vi "5-3Array_arrayoglu.vi"() -> ()   [LabVIEW 2024]
panel:
  out "max index(es)":i32[](array[numeric])
  out "max value 2":dbl
  out "transposed array":dbl[][](array[numeric])
  out "element 2":dbl
  in  "disabled index (col)":i32
  in  "index (row)":i32
  out "output array":dbl[](array[numeric])
  out "subarray":dbl[][](array[numeric])
  out "size(s) 2":i32[](array[numeric])
  in  "Array 8":dbl[][](array[numeric])
  out "Array 7":dbl[][](array[numeric])
  out "Array 6":dbl[](array[numeric])
  in  "length":i32
  in  "index 4":i32
  out "min value":i32
  out "max value":i32
  out "Array 5":dbl[](array[numeric])
  in  "new element/subarray 2":dbl
  in  "index 3":i32
  out "Array 4":dbl[](array[numeric])
  in  "new element/subarray":i32
  in  "index 2":i32
  in  "index":i32
  out "element":dbl
  out "size(s)":i32
  out "Array 3":dbl[](array[numeric])
  out "Array 2":dbl[](array[numeric])
  in  "dimension size":i32
  out "Array":dbl[](array[numeric])
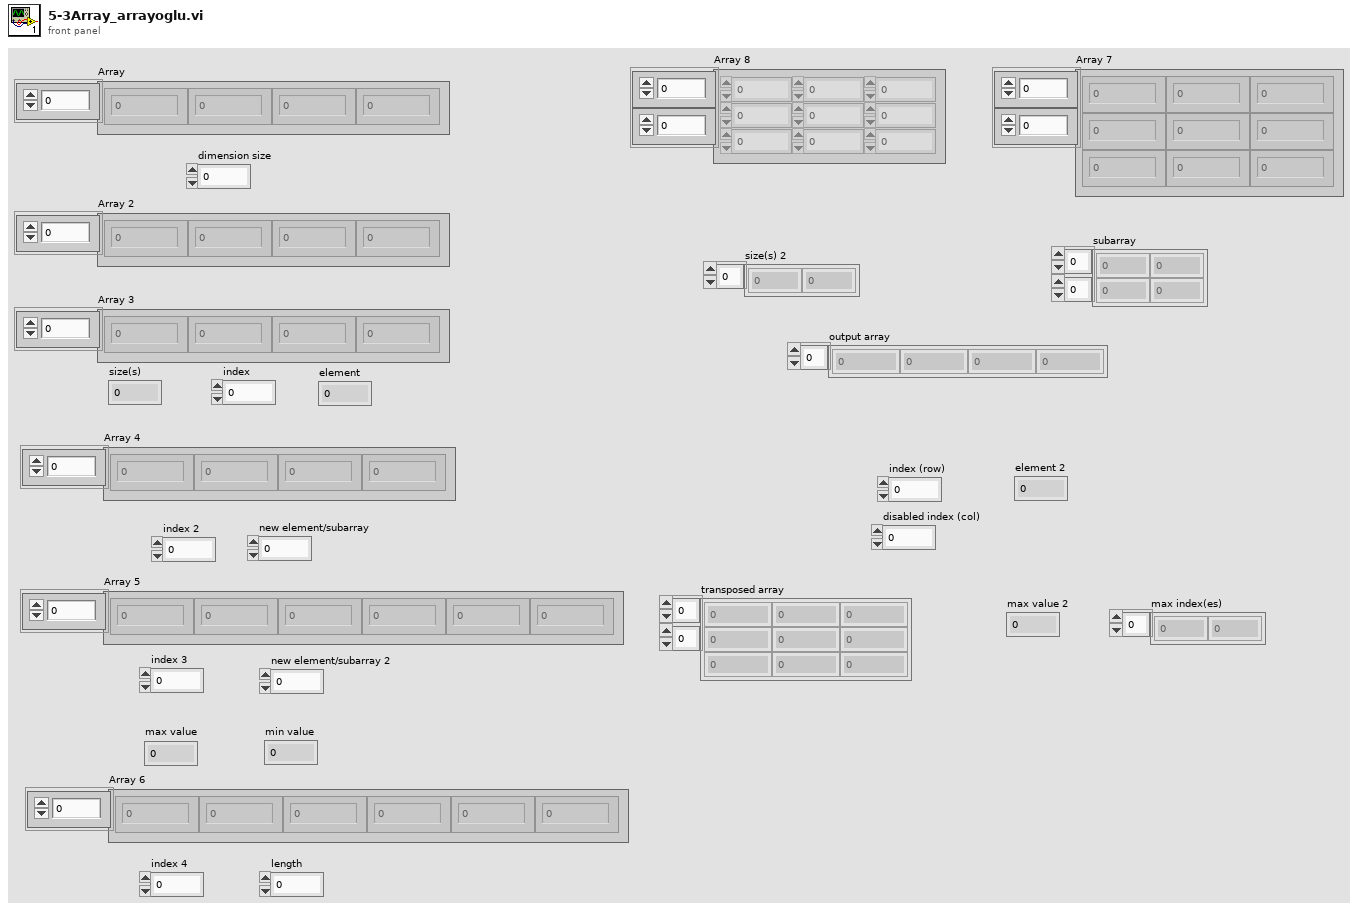
[diagram p1: front panel]
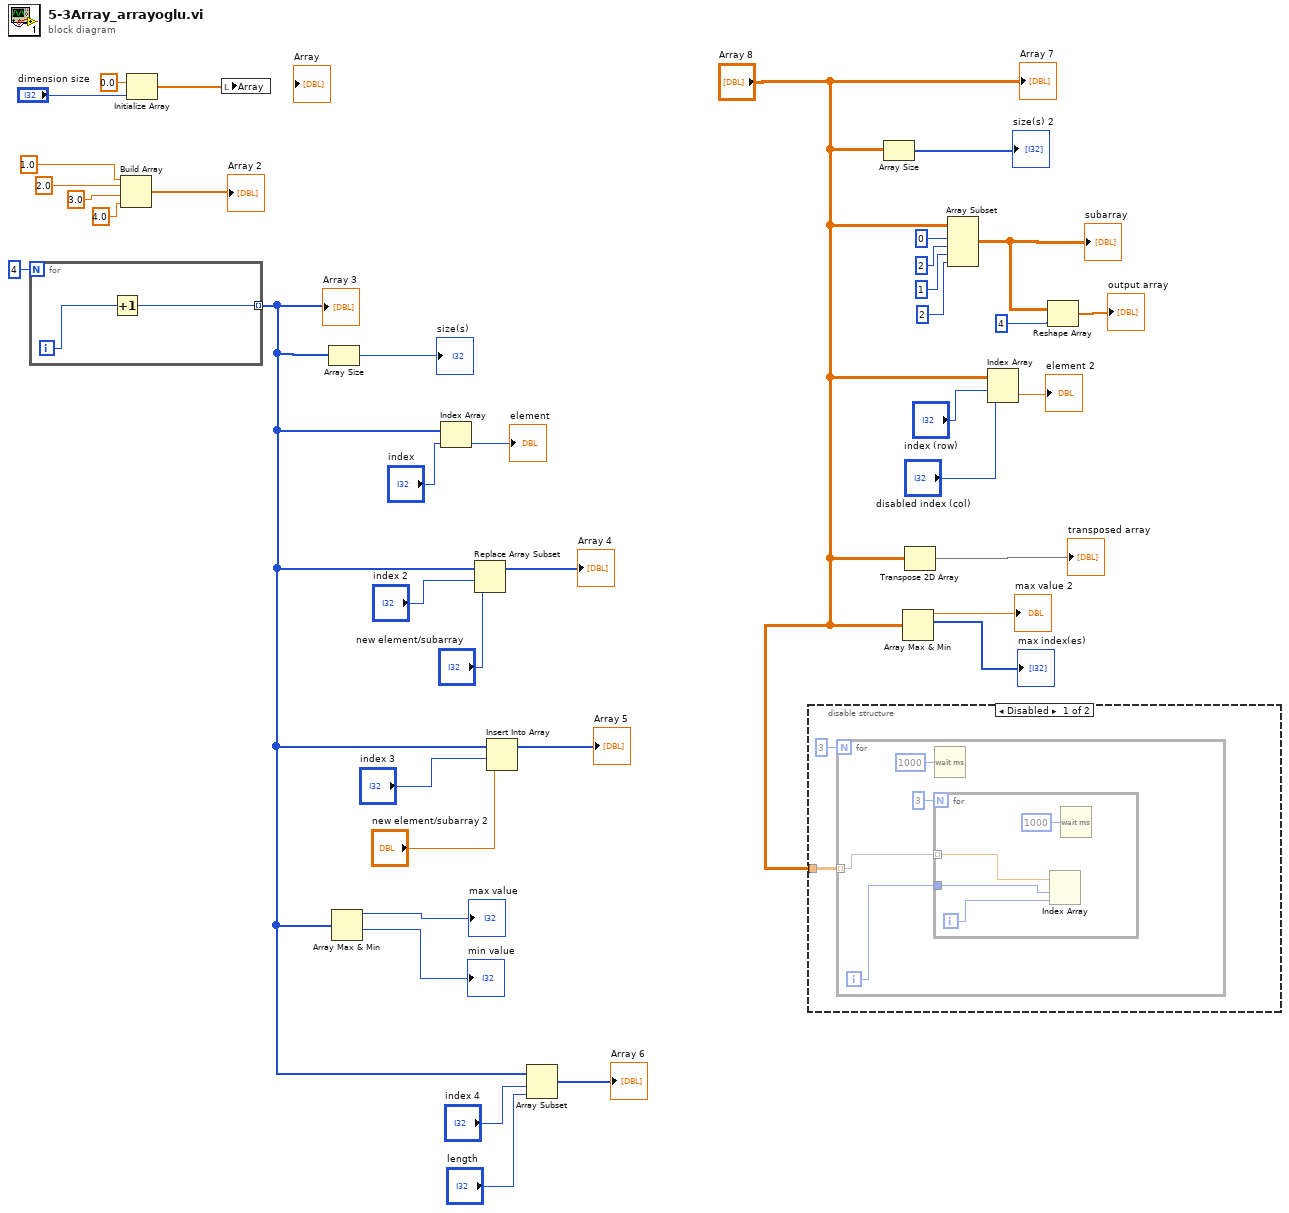
[diagram p0: block diagram]
diagram:
  n1 = for {
    N: 4 -> [_]
    tunnel: [w40] -> w36 mode=indexing
    i -> [w41]
    n2 = Increment(x=w41) -> (x+1=w40:i32)
  }
  "Array 3" <- w36
  n3 = Build Array "Build Array"(1.0 ("element"), 2.0 ("element"), 3.0 ("element"), 4.0 ("element")) -> (→"Array 2":dbl[])
  n4 = Initialize Array "Initialize Array"(0.0 ("element"), "dimension size") -> (w23:dbl[])
  n5 = local write "Array"(w23) -> ()
  n6 = Array Size(array=w36) -> (size(s)=→"size(s)":i32)
  n7 = Array Max & Min(array=w36) -> (max value=→"max value":i32, min value=→"min value":i32)  [unwired: 2 out]
  n8 = Index Array "Index Array"(array=w36, index="index") -> (element=→"element":i32)
  n9 = Replace Array Subset "Replace Array Subset"(array=w36, new element="new element/subarray", index="index 2") -> (→"Array 4":i32[])
  n10 = Insert Into Array "Insert Into Array"(array=w36, index="index 3", new element="new element/subarray 2") -> (→"Array 5":i32[])
  n11 = Array Subset "Array Subset"(array=w36, index="index 4", length="length") -> (→"Array 6":i32[])
  n12 = disable-structure shown="Disabled" {
    disable-tunnel: "Array 8" -> [w42 _]
    frame Disabled {
      n13 = for {
        N: 3 -> [_]
        tunnel: w42 -> [w45] mode=indexing
        i -> [w46]
        n14 = for {
          N: 3 -> [_]
          tunnel: w46 -> [w49]
          tunnel: w45 -> [w50] mode=indexing
          i -> [w48]
          n15 = Index Array "Index Array"(array=w50, index (row)=w49, index (col)=w48) -> ()  [unwired: 1 out]
          n16 = Wait (ms)(milliseconds to wait=u32 1000) -> ()  [unwired: 1 out]
        }
        n17 = Wait (ms)(milliseconds to wait=u32 1000) -> ()  [unwired: 1 out]
      }
    }
    frame Enabled {
    }
  }
  n18 = Array Size(array="Array 8") -> (size(s)=→"size(s) 2":i32[])
  n19 = Array Max & Min(array="Array 8") -> (max value=→"max value 2":dbl, max index (indices)=→"max index(es)":i32[])  [unwired: 2 out]
  n20 = Transpose 2D Array(2D array="Array 8") -> (transposed array=→"transposed array":dbl[][])
  n21 = Array Subset "Array Subset"(array="Array 8", index (row)=0 ("index"), length (row)=2 ("index"), index (col)=1 ("index"), length (col)=2 ("length")) -> (w10:dbl[][])
  "subarray" <- w10
  n22 = Index Array "Index Array"(array="Array 8", index (row)="index (row)", index (col)="disabled index (col)") -> (element=→"element 2":dbl)
  n23 = Reshape Array "Reshape Array"(w10, 4 ("dimension size")) -> (→"output array":dbl[])
  "Array 7" <- "Array 8"
